vi "Write Connected IPAddress.vi"(8 "error in (no error)":errorcluster, 10 "Connected IPAddress":u32, 11 "Receiver in":refnum<class "Receiver.lvclass">) -> (0 "error out":errorcluster, 3 "Receiver out":refnum<class "Receiver.lvclass">)   [LabVIEW 2013, in "Receiver.lvlib" / "Receiver.lvclass"]
uses:
  Receiver.lvclass
  Receiver.lvclass/Receiver.ctl
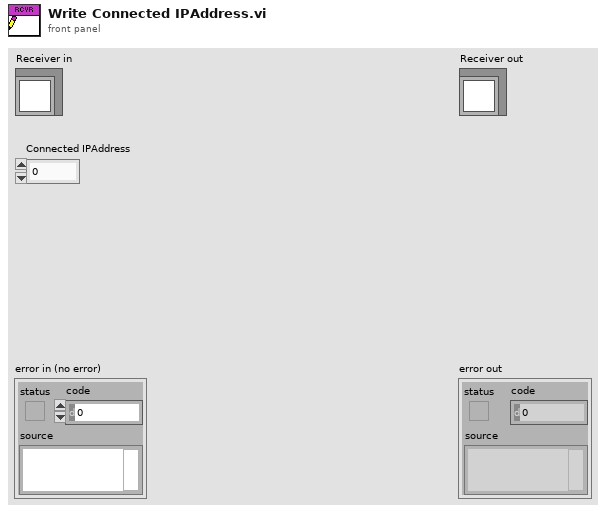
[diagram p1: front panel]
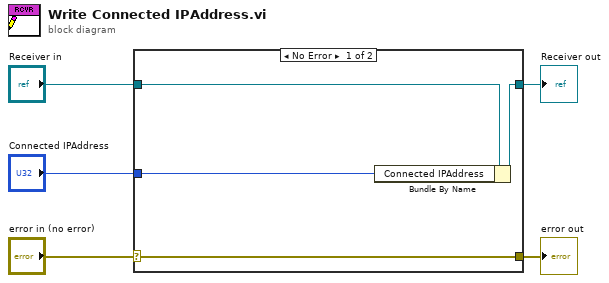
[diagram p0: block diagram]
diagram:
  n1 = case shown="No Error" "error in (no error)" {
    selector: "error in (no error)" -> [w9 w10]
    tunnel: [w9 w10] -> w4
    tunnel: [w7 w11] -> w2
    tunnel: "Receiver in" -> [w8 w11]
    tunnel: "Connected IPAddress" -> [w6 _]
    frame No Error {
      n2 = Bundle By Name(cluster=w8, "Connected IPAddress"=w6) -> (w7:refnum<class "Receiver.lvclass">)
    }
    frame Error {
    }
  }
  "error out" <- w4
  "Receiver out" <- w2
